vi "Destroy.vi"(8 "error in (no error)":errorcluster, 11 "Trajectory Drawer in":refnum<class "Trajectory Drawer.lvclass">) -> (0 "error out":errorcluster, 2 "Root Ref.":refnum<vi>, 3 "Trajectory Drawer out":refnum<class "Trajectory Drawer.lvclass">)   [LabVIEW 2014, in "Trajectory Drawer.lvclass"]
uses:
  Trajectory Drawer.lvclass
  <vilib>/Utility/miscctls.llb/LVRGBAColorTypeDef.ctl
  Trajectory Drawer.lvclass/Trajectory Drawer.ctl
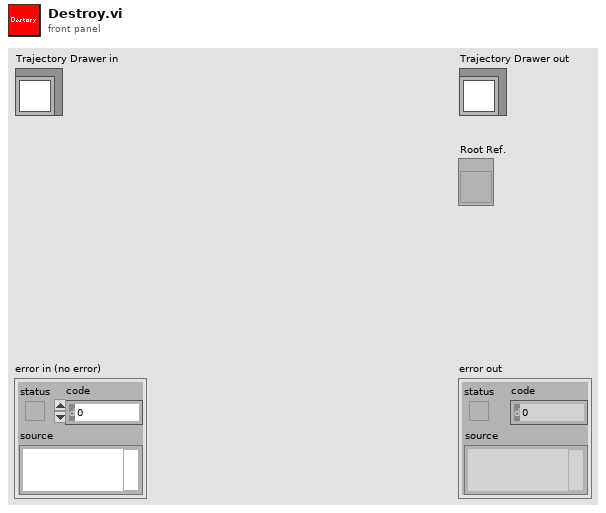
[diagram p1: front panel]
types:
  T1 = typedef "LVRGBAColorTypeDef.ctl" = cluster{"Red":sgl, "Green":sgl, "Blue":sgl, "Alpha":sgl}
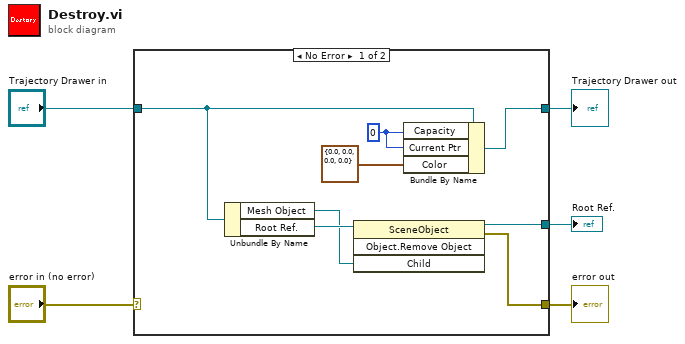
[diagram p0: block diagram]
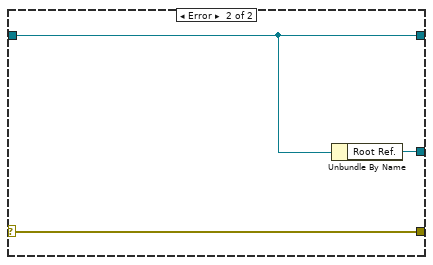
[diagram p2: hidden frame]
diagram:
  n1 = case shown="No Error" "error in (no error)" {
    selector: "error in (no error)" -> [_ w16]
    tunnel: [w6 w16] -> w4
    tunnel: [w12 w15] -> w2
    tunnel: "Trajectory Drawer in" -> [w13 w15]
    tunnel: [w7 w14] -> w1
    frame No Error {
      w11 = 0
      n2 = Unbundle By Name(w13) -> ("Mesh Object"=w8:refnum<vi>, "Root Ref."=w9:refnum<vi>)
      n3 = invoke class="SceneObject" method="Object.Remove Object"(reference=w9, "Child"=w8) -> (reference out=w7:refnum<vi>, error out=w6:errorcluster)  [unwired: 2 in, 2 out]
      n4 = Bundle By Name(cluster=w13, "Capacity"=w11, "Current Ptr"=w11, "Color"=T1 {"Red"=0.0, "Green"=0.0, "Blue"=0.0, "Alpha"=0.0}) -> (w12:refnum<class "Trajectory Drawer.lvclass">)
    }
    frame Error {
      n5 = Unbundle By Name(w15) -> ("Root Ref."=w14:refnum<vi>)
    }
  }
  "error out" <- w4
  "Trajectory Drawer out" <- w2
  "Root Ref." <- w1
